vi "FolderMon Get Folder Listing.vi"(8 "error in (no error)":errorcluster, 11 "Path":path) -> (0 "error out":errorcluster, 2 "file names":string[](array[string]), 3 "path out":path)   [LabVIEW 2011]
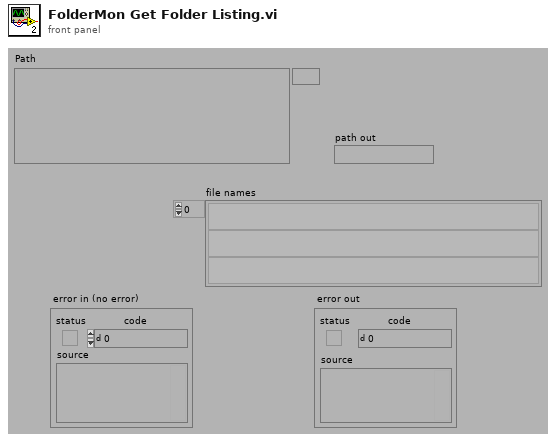
[diagram p1: front panel]
types:
  T1 = enum32{"invalid app kind", "Development System", "Run Time System", "Student Edition", "Embedded LabVIEW", "Evaluation", "Custom"}
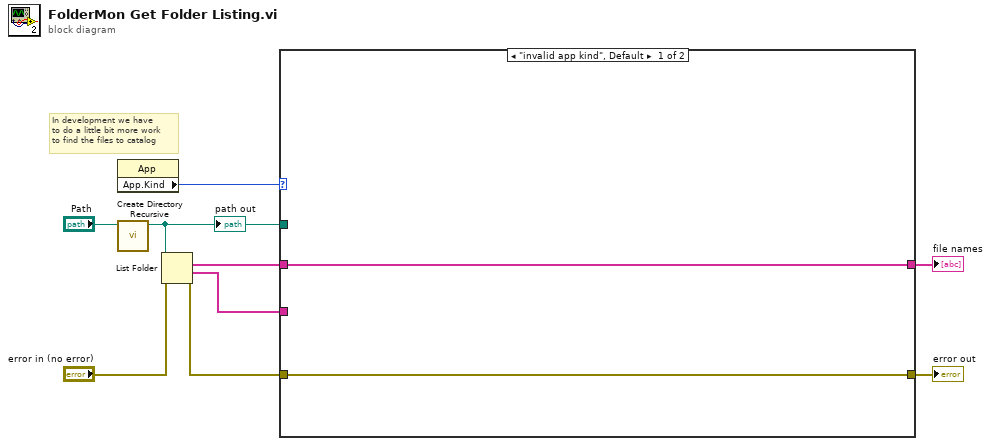
[diagram p0: block diagram]
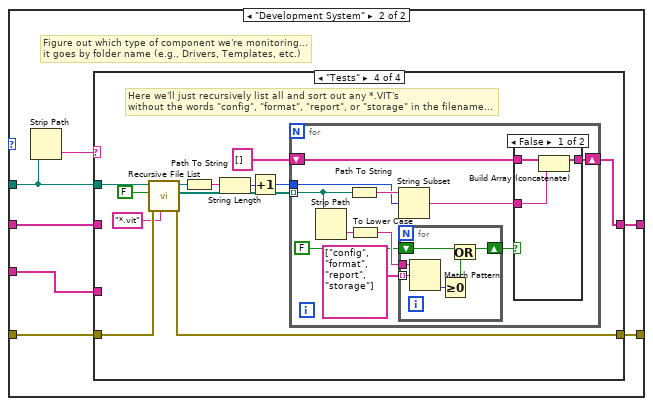
[diagram p2: hidden frame]
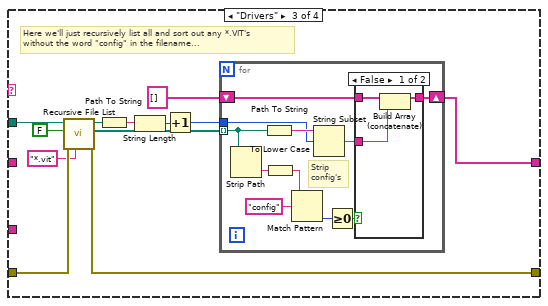
[diagram p5: hidden frame]
diagram:
  # "In development we have\nto do a little bit more work\nto find the files to catalog"
  n1 = property class="App"() -> ("App.Kind"=w9:T1)  [unwired: 2 in, 2 out]
  n2 = call <vilib>:"Create Directory Recursive.vi"("directory"="Path") -> ("directory copy"=w1:path)  [unwired: 2 in, 4 out]
  "path out" <- w1
  n3 = List Folder(path=w1, error in="error in (no error)") -> (filenames=w4:string[], folder names=w3:string[], error out=w7:errorcluster)  [unwired: 3 out]
  n4 = case shown="\"invalid app kind\", Default" w9 {
    tunnel: w7 -> [w11 w13]
    tunnel: [w11 w12] -> w6
    tunnel: [w10 w14] -> w5
    tunnel: w4 -> [w10 w15]
    tunnel: w3 -> [_ w16]
    tunnel: w1 -> [_ w17]
    frame "invalid app kind", Default {
    }
    frame "Development System" {
      # "Figure out which type of component we're monitoring...\nit goes by folder name (e.g., Drivers, Templates, etc.)"
      n5 = Strip Path(path=w17) -> (name=w18:string)  [unwired: 1 out]
      n6 = case shown="\"Tests\"" w18 {
        tunnel: w17 -> [_ _ w34 w61]
        tunnel: w16 -> [_ _ _ _]
        tunnel: w15 -> [w20 w22 _ _]
        tunnel: [w20 w22 w27 w54] -> w14
        tunnel: w13 -> [w19 w21 w32 w59]
        tunnel: [w19 w21 w30 w57] -> w12
        frame "UNKNOWN", Default {
          # "Have to punt here - don't\nknow what we're looking for\nso fall back on the default\nbehavior..."
        }
        frame "Templates" {
          # "Templates follow the standard\nmonitoring convention regardless\nof App.Kind..."
        }
        frame "Drivers" {
          # "Here we'll just recursively list all and sort out any *.VIT's\nwithout the word \"config\" in the filename..."
          n7 = call <vilib>:"Recursive File List.vi"("pattern"="*.vit", "error in (no error)"=w32, "Treat LLBs as Folders?"=FALSE, "Folder Path"=w34) -> ("error out"=w30:errorcluster, "All Files in Dir"=w29:path[], "dup Folder Path"=w26:path)  [unwired: 5 out]
          n8 = Path To String(path=w26) -> (string=w25:string)
          n9 = String Length(string=w25) -> (length=w24:i32)
          n10 = Increment(x=w24) -> (x+1=w23:i32)
          n11 = for {
            tunnel: w29 -> [w38] mode=indexing
            shift-right: [w40] -> w27
            shift-left: string[] [] ("folder names") -> [w41]
            tunnel: w23 -> [w36]
            # "Strip\nconfig's"
            n12 = Strip Path(path=w38) -> (name=w39:string)  [unwired: 1 out]
            n13 = Path To String(path=w38) -> (string=w37:string)
            n14 = To Lower Case(string=w39) -> (all lower case string=w44:string)
            n15 = Match Pattern(string=w44, regular expression="config") -> (offset past match=w43:i32)  [unwired: 4 out]
            n16 = String Subset(string=w37, offset (0)=w36) -> (substring=w35:string)  [unwired: 1 out]
            n17 = Greater Or Equal To 0?(x=w43) -> (x >= 0?=w42:bool)
            n18 = case shown="False" w42 {
              tunnel: w41 -> [w48 w49]
              tunnel: [w47 w49] -> w40
              tunnel: w35 -> [w46 _]
              frame False {
                n19 = Build Array (concatenate)(w48, w46) -> (w47:string[])
              }
              frame True {
              }
            }
          }
        }
        frame "Tests" {
          # "Here we'll just recursively list all and sort out any *.VIT's\nwithout the words \"config\", \"format\", \"report\", or \"storage\" in the filename..."
          n20 = call <vilib>:"Recursive File List.vi"("pattern"="*.vit", "error in (no error)"=w59, "Treat LLBs as Folders?"=FALSE, "Folder Path"=w61) -> ("error out"=w57:errorcluster, "All Files in Dir"=w56:path[], "dup Folder Path"=w53:path)  [unwired: 5 out]
          n21 = Path To String(path=w53) -> (string=w52:string)
          n22 = String Length(string=w52) -> (length=w51:i32)
          n23 = Increment(x=w51) -> (x+1=w50:i32)
          n24 = for {
            tunnel: w56 -> [w69] mode=indexing
            shift-right: [w71] -> w54
            shift-left: string[] [] ("folder names") -> [w72]
            tunnel: w50 -> [w67]
            n25 = Strip Path(path=w69) -> (name=w70:string)  [unwired: 1 out]
            n26 = Path To String(path=w69) -> (string=w68:string)
            n27 = To Lower Case(string=w70) -> (all lower case string=w64:string)
            n28 = String Subset(string=w68, offset (0)=w67) -> (substring=w66:string)  [unwired: 1 out]
            n29 = for {
              shift-right: [w76] -> w62
              shift-left: FALSE -> [w75]
              tunnel: string[] ["config", "format", "report", "storage"] ("folder names") -> [w74] mode=indexing
              tunnel: w64 -> [w73]
              n30 = Match Pattern(string=w73, regular expression=w74) -> (offset past match=w78:i32)  [unwired: 4 out]
              n31 = Greater Or Equal To 0?(x=w78) -> (x >= 0?=w77:bool)
              n32 = Or(x=w75, y=w77) -> (x .or. y?=w76:bool)
            }
            n33 = case shown="False" w62 {
              tunnel: w72 -> [w81 w82]
              tunnel: [w80 w82] -> w71
              tunnel: w66 -> [w79 _]
              frame False {
                n34 = Build Array (concatenate)(w81, w79) -> (w80:string[])
              }
              frame True {
              }
            }
          }
        }
      }
    }
  }
  "error out" <- w6
  "file names" <- w5
